vi "Get_picture_size.vi"(7 "DDAS  (W = 400, H = 300)":T1={"Width"=400, "Height"=300}, 8 "error in (no error)":errorcluster, 10 "image data":T2) -> (0 "error out":errorcluster, 2 "Draw Area Size":T1)   [LabVIEW 2020]
doc: "This VI takes <b>#typedef image data</b> and returns cluster <b>#typedef Draw Area Size </b> which contains <b>Width</b> and <b>Height</b> of the input image. If output cluster <b>Draw Area Size</b> elements: <b>Width</b> and <b>Height</b> are eqaul to 0, then it is reinitialize to <b>Default Draw Area Size</b>."
uses:
  <vilib>/Utility/miscctls.llb/LVBoundsTypeDef.ctl
  <vilib>/picture/picture.llb/imagedata.ctl
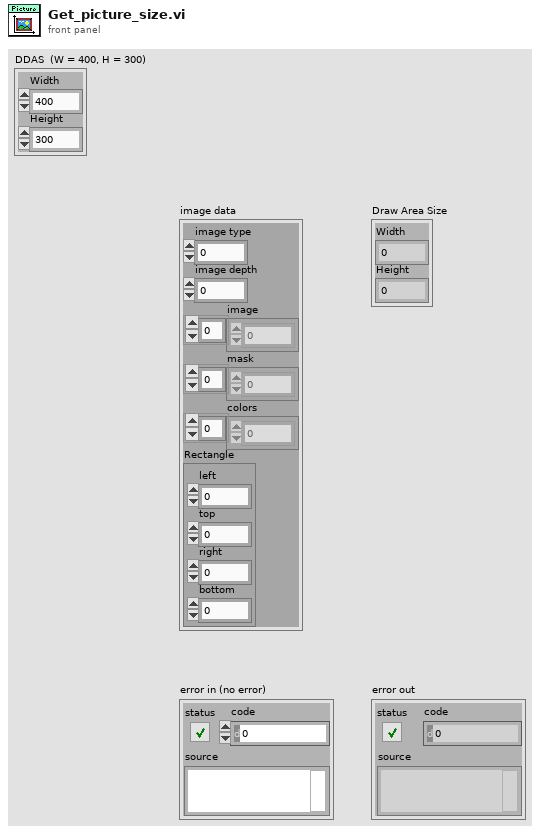
[diagram p1: front panel]
types:
  T1 = typedef "LVBoundsTypeDef.ctl" = cluster{"Width":u32, "Height":u32}
  T2 = typedef "imagedata.ctl" = cluster{"image type":i32, "image depth":i32, "image":u8[], "mask":u8[], "colors":u32[], "Rectangle":cluster{"left":i16, "top":i16, "right":i16, "bottom":i16}}
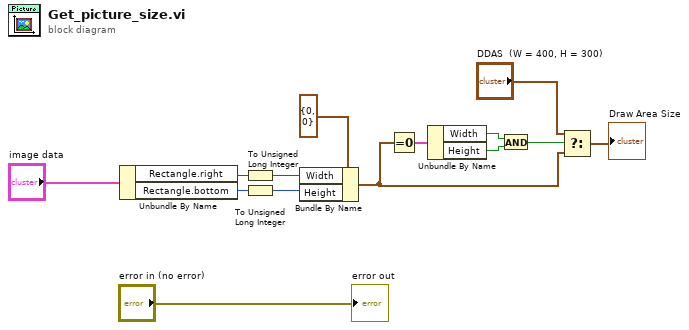
[diagram p0: block diagram]
diagram:
  n1 = Unbundle By Name("image data") -> ("Rectangle.right"=w10:i16, "Rectangle.bottom"=w11:i16)
  n2 = To Unsigned Long Integer(number=w10) -> (unsigned 32bit integer=w12:u32)
  n3 = To Unsigned Long Integer(number=w11) -> (unsigned 32bit integer=w13:u32)
  n4 = Bundle By Name(cluster=T1 {"Width"=0, "Height"=0} ("Draw Area Size"), "Width"=w12, "Height"=w13) -> (w3:T1)
  n5 = Equal To 0?(x=w3) -> (x = 0?=w7:cluster{"Width":bool, "Height":bool})
  n6 = Unbundle By Name(w7) -> ("Width"=w6:bool, "Height"=w5:bool)
  n7 = And(x=w6, y=w5) -> (x .and. y?=w4:bool)
  n8 = Select(t="DDAS  (W = 400, H = 300)", s=w4, f=w3) -> (s? t:f=→"Draw Area Size":T1)
  "error out" <- "error in (no error)"
